vi "Coord window-Settings window.vi"() -> (3 "Cancelled?":bool)   [LabVIEW 2020]
doc: "Use this template to create a dialog box with event handling."
uses:
  Globals/Coord window-Globals.vi
  Global Variables/General Globals.vi
panel:
  in  "Motor dot size":enum16{"Tiny", "Normal", "Medium", "Large"}(ring)
  in  "Motor coordinates colour":u32(colorbox)=6618880
  in  "OK":bool
  # "Settings"
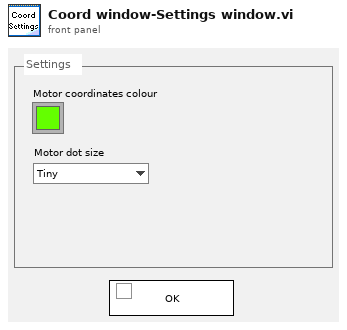
[diagram p1: front panel]
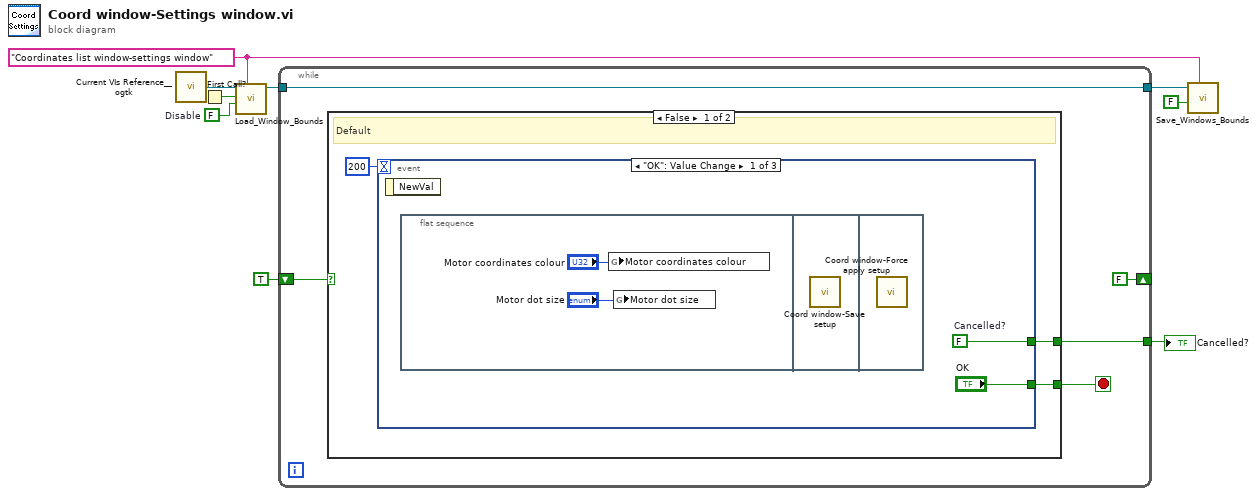
[diagram p0: block diagram]
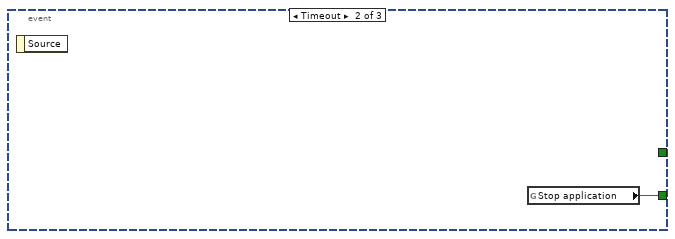
[diagram p2: hidden frame]
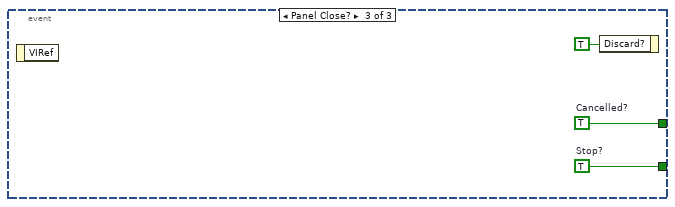
[diagram p3: hidden frame]
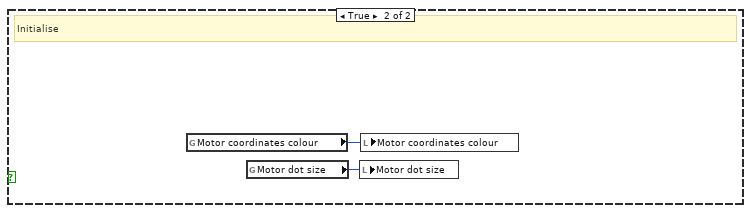
[diagram p4: hidden frame]
diagram:
  w5 = FALSE  # Disable
  w4 = "Coordinates list window-settings window" ("Window Name (i.e. Key)")
  n1 = call <userlib>:"Current VIs Reference__ogtk.vi"() -> ("Current VI's reference"=w7:refnum<vi>)  [unwired: 5 in]
  n2 = First Call?() -> (First Call?: T/F=w6:bool)
  n3 = call "Load_Window_Bounds.vi"("Window Name (i.e. Key)"=w4, "Disable"=w5, "First Call"=w6, "Window VI's Ref"=w7) -> ("reference out"=w2:refnum<vi>)  [unwired: 4 in, 3 out]
  n4 = while {
    tunnel: [w13] -> w9
    shift-right: [FALSE] -> _
    shift-left: TRUE -> [w12]
    tunnel: w2 -> [w10]
    tunnel: [w10] -> w1
    stop <- w14 stop-if-true
    n5 = case shown="False" w12 {
      tunnel: [w17 _] -> w14
      tunnel: [w16 _] -> w13
      frame False {
        # "Default"
        n6 = event shown="[0] \"OK\": Value Change" {
          selector: _ -> [_ _ _]
          dyn-events: _ -> [_ _ _]
          timeout: 200 -> [_ _ _]
          tunnel: ["OK" w22 w24] -> w17
          tunnel: [w19 _ w23] -> w16
          event "OK": Value Change {
            w19 = FALSE  # Cancelled?
            n7 = event-data() -> ()  [unwired: 1 in, 1 out]
            n8 = flat-sequence {
              frame #0 {
                n9 = global write "Coord window-Globals.vi" "Motor coordinates colour"("Motor coordinates colour") -> ()
                n10 = global write "Coord window-Globals.vi" "Motor dot size"("Motor dot size") -> ()
              }
              frame #1 {
                n11 = call "Coord window-Save setup.vi"() -> ()  [unwired: 11 in, 1 out]
              }
              frame #2 {
                n12 = call "Coord window-Force apply setup.vi"() -> ()  [unwired: 12 in]
              }
            }
          }
          event Timeout {
            n13 = event-data() -> ()  [unwired: 1 in, 1 out]
            n14 = global read "General Globals.vi" "Stop application"() -> (w22:bool)
          }
          event Panel Close? {
            w23 = TRUE  # Cancelled?
            w24 = TRUE  # Stop?
            n15 = event-data() -> ()  [unwired: 1 in, 1 out]
            n16 = event-data("Discard?"=TRUE) -> ()  [unwired: 1 in, 1 out]
          }
        }
      }
      frame True {
        # "Initialise"
        n17 = global read "Coord window-Globals.vi" "Motor coordinates colour"() -> (w27:u32)
        n18 = global read "Coord window-Globals.vi" "Motor dot size"() -> (w26:i16)
        n19 = local write "Motor dot size"(w26) -> ()
        n20 = local write "Motor coordinates colour"(w27) -> ()
      }
    }
  }
  "Cancelled?" <- w9
  n21 = call "Save_Windows_Bounds.vi"("Window Name (i.e. Key)"=w4, "Front Panel Window:Open"=FALSE, "Window VI's Ref"=w1) -> ()  [unwired: 8 in, 1 out]
